vi "Assert String Not Contains String Ignoring Case.vi"(5 "Needle":string, 7 "Message (\"\")":string, 8 "error in (no error)":errorcluster, 10 "Haystack":string) -> (0 "error out":errorcluster)   [LabVIEW 2017, in "Transparent Assertions.lvlib"]
doc: "Asserts that a string does not contain the expected substring, ignoring case differences. Returns an error if the assertion fails, and optionally appends a custom message to the error."
uses:
  Transparent Assertions.lvlib
  LogicalNot/LogicalNot.lvclass
  StringContains/StringContains.lvclass
  C:/Users/pasca/Projects/Home/TransparentAssertions/src/Transparent Assertions/Constraints/Constraint/Constraint.lvclass
  UnaryOperator/UnaryOperator.lvclass
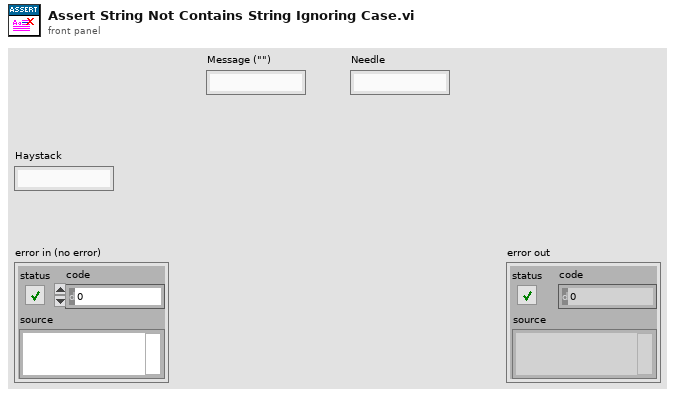
[diagram p1: front panel]
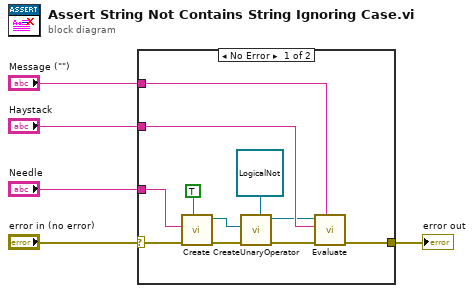
[diagram p0: block diagram]
diagram:
  n1 = case shown="No Error" "error in (no error)" {
    selector: "error in (no error)" -> [w12 w17]
    tunnel: "Haystack" -> [w15 _]
    tunnel: [w14 w17] -> w4
    tunnel: "Message (\"\")" -> [w13 _]
    tunnel: "Needle" -> [w11 _]
    frame No Error {
      n2 = call "Create.vi"("Ignore Case (F)"=TRUE, "error in (no error)"=w12, "Needle"=w11) -> ("error out"=w16:errorcluster, "StringContains"=w8:refnum<class "StringContains.lvclass">)  [unwired: 7 in]
      n3 = call-dynamic "CreateUnaryOperator.vi"("UnaryOperator In"=refnum<class "LogicalNot.lvclass"> refnum ("Constraint.lvlib:LogicalNot.lvclass"), "error in (no error)"=w16, "Constraint"=w8) -> ("error out"=w9:errorcluster, "UnaryOperator"=w7:refnum<class "UnaryOperator.lvclass">)  [unwired: 7 in]
      n4 = call-dynamic "Evaluate.vi"("Message (\"\")"=w13, "error in (no error)"=w9, "Actual"=w15, "Constraint in"=w7) -> ("error out"=w14:errorcluster)  [unwired: 6 in, 1 out]
    }
    frame Error {
    }
  }
  "error out" <- w4
